vi "SUB_Password_keyin.vi"() -> (1 "Pass?":bool)   [LabVIEW 2011]
uses:
  <vilib>/event_ctls.llb/eventvkey.ctl
  Instance           1 26Saved   SUB_Password_keyin .vi
panel:
  out "軟體版本Software Version":string
  in  "Password":string="192.168.1.3\n192.168.1.1\n192.168.1.1"
  # "Input the Password\n輸入授權密碼.請TE依實際狀況修改"
  # "注意:未依照規範,亂改會造成測試NG\nDon't abuse this tool for too loose tolerance"
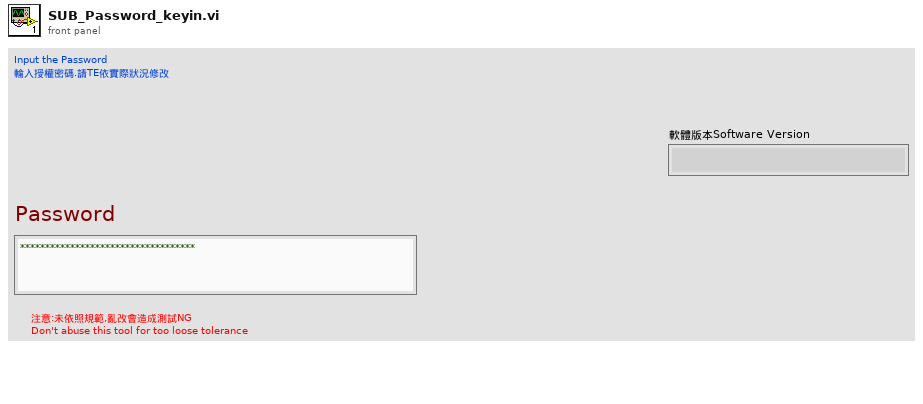
[diagram p1: front panel]
types:
  T1 = typedef "eventvkey.ctl" = enum16{"ASCII", "Enter", "Return", "Shift", "Ctrl", "Alt", "Cmd", "Opt", "Caps", "NumLock", "Clear", "Break", "Up", "Down", "Left", "Right", "Insert", "Delete", "Home", "End", "PageUp", "PageDown", "Escape", "Help", "Pause", "ScrollLock", "F1", "F2", "F3", "F4", "F5", "F6", "F7", "F8", "F9", "F10", "F11", "F12", "F13", "F14", "F15", "F16", "F17", "F18", "F19", "F20", "F21", "F22", "F23", "F24", "Play", "VolumeUp", "VolumeDown", "Mute", "Two Byte Char"}
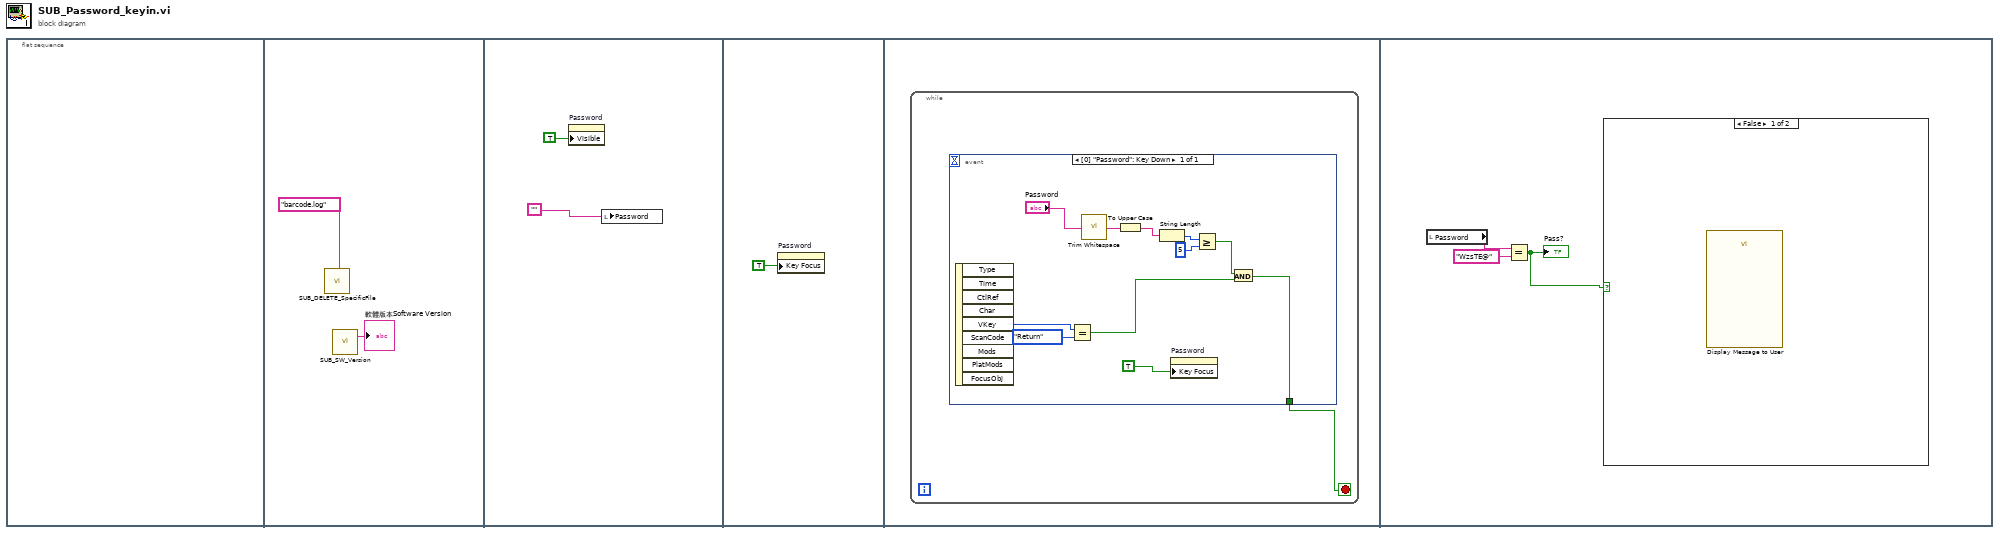
[diagram p0: block diagram]
diagram:
  n1 = flat-sequence {
    frame #0 {
    }
    frame #1 {
      n2 = call "SUB_DELETE_SpecificFile.vi"("Filename to be  Deleted"="barcode.log" ("Filename")) -> ()  [unwired: 2 in, 1 out]
      n3 = call "SUB_SW_Version.vi"() -> ("Current Software Version"=→"軟體版本Software Version":string)  [unwired: 3 in]
    }
    frame #2 {
      n4 = property on="Password" class="Str"("Visible"=TRUE) -> ()  [unwired: 2 in, 2 out]
      n5 = local write "Password"("") -> ()
    }
    frame #3 {
      n6 = property on="Password" class="Str"("Key Focus"=TRUE) -> ()  [unwired: 2 in, 2 out]
    }
    frame #4 {
      n7 = while {
        stop <- w6 stop-if-true
        n8 = event shown="[0] \"Password\": Key Down" {
          selector: _ -> [_]
          dyn-events: _ -> [_]
          timeout: _ -> [_]
          tunnel: [w8] -> w6
          event "Password": Key Down {
            n9 = event-data() -> ("VKey"=w11:T1)  [unwired: 1 in, 8 out]
            n10 = Equal?(x=w11, y=eventvkey."Return") -> (x = y?=w9:bool)
            n11 = call <vilib>:"Trim Whitespace.vi"("string"="Password") -> ("trimmed string"=w14:string)  [unwired: 1 in]
            n12 = To Upper Case(1:w14) -> (0:w13:string)
            n13 = String Length(string=w13) -> (length=w17:i32)
            n14 = property on="Password" class="Str"("Key Focus"=TRUE) -> ()  [unwired: 2 in, 2 out]
            n15 = Greater Or Equal?(x=w17, y=5) -> (x >= y?=w15:bool)
            n16 = And(x=w15, y=w9) -> (x .and. y?=w8:bool)
          }
        }
      }
    }
    frame #5 {
      n17 = local read "Password"() -> (w20:string)
      n18 = Equal?(x=w20, y="WzsTE@") -> (x = y?=w18:bool)
      "Pass?" <- w18
      n19 = case shown="False" w18 {
        frame False {
          n20 = call "Display Message to User"() -> ()  [unwired: 10 in, 2 out]
        }
        frame True {
        }
      }
    }
  }
